vi "CloseState.vi"(8 "Error In":errorcluster, 11 "Queue In":refnum<queue>) -> (0 "Error Out":errorcluster)   [LabVIEW 2010]
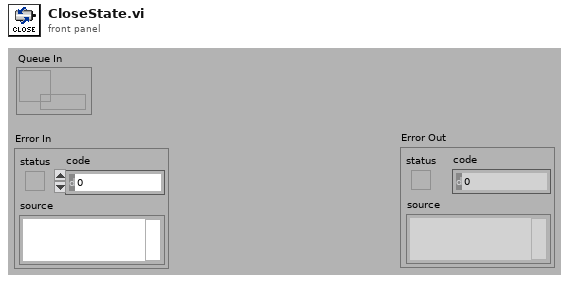
[diagram p1: front panel]
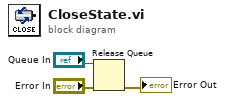
[diagram p0: block diagram]
diagram:
  n1 = Release Queue(queue="Queue In", error in (no error)="Error In") -> (error out=→"Error Out":errorcluster)  [unwired: 1 in, 2 out]
